vi "Pre Launch Init.vi"(11 "Nested in":refnum<class "Messages Actor.lvclass">) -> (0 "error out":errorcluster, 3 "Nested out":refnum<class "Messages Actor.lvclass">)   [LabVIEW 2020, in "Messages Actor.lvlib" / "Messages Actor.lvclass"]
doc: "(<B>Filename</B>: Actor Framework.lvlib:Actor.lvclass:Pre Launch Init.vi)\n\nDefines behavior that occurs after the Launch Nested Actor method is invoked but before the actor's Actor Core method begins running.\n\nBy default, this method does nothing. A descendant class may override it to define behavior."
uses:
  Messages Actor.lvclass
  C:/Program Files (x86)/National Instruments/LabVIEW 2020/vi.lib/ActorFramework/Actor/Actor.lvclass
  Controls/Language Enum.ctl
  Messages Actor.lvclass/Messages Actor.ctl
  <vilib>/ActorFramework/Actor/Actor.lvclass/Actor.ctl
  <vilib>/ActorFramework/Message Enqueuer/Message Enqueuer.lvclass/Message Enqueuer.ctl
  <vilib>/ActorFramework/Message Enqueuer/Enqueue.vi
  <vilib>/ActorFramework/Message Enqueuer/Init from Existing Queue.vi
  Messages Actor Messages/Initialization Msg/Initialization Msg.lvclass
  C:/Program Files (x86)/National Instruments/LabVIEW 2020/vi.lib/ActorFramework/Message/Message.lvclass
  Messages Actor Messages/UpdateLanguage Msg/UpdateLanguage Msg.lvclass
  <vilib>/ActorFramework/Message Priority Queue/Priority Enqueue.vi
  <vilib>/ActorFramework/Message Enqueuer/Message Enqueuer.lvclass
  <vilib>/ActorFramework/Actor/Actor.lvclass
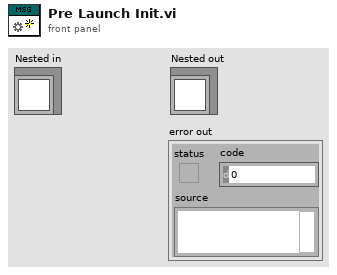
[diagram p1: front panel]
types:
  T1 = typedef "Language Enum.ctl" = enum16{"English", "Español", "Français"}
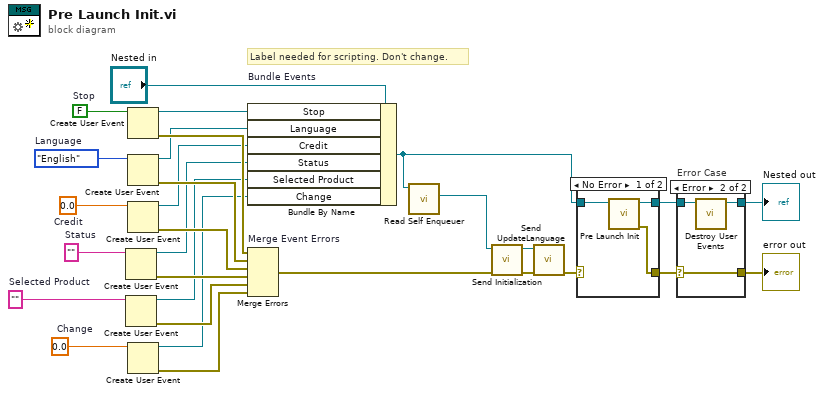
[diagram p0: block diagram]
diagram:
  w3 = 0.0  # Change
  w6 = ""  # Selected Product
  w9 = ""  # Status
  w12 = 0.0  # Credit
  w21 = Language_Enum."English"  # Language
  w28 = FALSE  # Stop
  # "Label needed for scripting. Don't change."
  n1 = Create User Event(user event datatype=w9) -> (user event=w8:refnum<user-event>, error out=w7:errorcluster)  [unwired: 1 in]
  n2 = Create User Event(user event datatype=w6) -> (user event=w5:refnum<user-event>, error out=w4:errorcluster)  [unwired: 1 in]
  n3 = Create User Event(user event datatype=w28) -> (user event=w25:refnum<user-event>, error out=w27:errorcluster)  [unwired: 1 in]
  n4 = Create User Event(user event datatype=w21) -> (user event=w20:refnum<user-event>, error out=w19:errorcluster)  [unwired: 1 in]
  n5 = Create User Event(user event datatype=w12) -> (user event=w11:refnum<user-event>, error out=w10:errorcluster)  [unwired: 1 in]
  n6 = Create User Event(user event datatype=w3) -> (user event=w2:refnum<user-event>, error out=w1:errorcluster)  [unwired: 1 in]
  n7 = Bundle By Name "Bundle Events"(cluster="Nested in", "Stop"=w25, "Language"=w20, "Credit"=w11, "Status"=w8, "Selected Product"=w5, "Change"=w2) -> (w18:refnum<class "Messages Actor.lvclass">)
  n8 = Merge Errors "Merge Event Errors"(w27, w19, w10, w7, w4, w1) -> (w15:errorcluster)
  n9 = call <vilib>:"Read Self Enqueuer.vi"("Actor"=w18) -> ("Self Enqueuer"=w14:refnum<class "Message Enqueuer.lvclass">)  [unwired: 10 in]
  n10 = call "Send Initialization.vi"("error in (no error)"=w15, "Message Enqueuer"=w14) -> ("error out"=w16:errorcluster, "Message Enqueuer out"=w13:refnum<class "Message Enqueuer.lvclass">)  [unwired: 8 in]
  n11 = call "Send UpdateLanguage.vi"("error in (no error)"=w16, "Message Enqueuer"=w13) -> ("error out"=w17:errorcluster)  [unwired: 8 in, 1 out]
  n12 = case shown="No Error" w17 {
    selector: w17 -> [_ w34]
    tunnel: [w32 w33] -> w23
    tunnel: w18 -> [w31 w33]
    tunnel: [w30 w34] -> w22
    frame No Error {
      n13 = call-parent "Pre Launch Init.vi"("Actor in"=w31) -> ("error out"=w30:errorcluster, "Actor out"=w32:refnum<class "Messages Actor.lvclass">)  [unwired: 9 in]
    }
    frame Error {
    }
  }
  n14 = case "Error Case" shown="Error" w22 {
    selector: w22 -> [w35 w39]
    tunnel: w23 -> [w36 w38]
    tunnel: [w36 w37] -> w26
    tunnel: [w35 w39] -> w24
    frame No Error {
    }
    frame Error {
      n15 = call "Destroy User Events.vi"("UI Template in"=w38) -> ("UI Template out"=w37:refnum<class "Messages Actor.lvclass">)  [unwired: 10 in]
    }
  }
  "error out" <- w24
  "Nested out" <- w26
